vi "Comparison and boolean.VI"() -> ()   [LabVIEW 2019]
panel:
  out "result":bool
  in  "num 3":dbl=20.0
  out "result":bool
  in  "num2":dbl
  out "result":bool
  in  "num 1":dbl=20.0
  out "result":bool
  in  "boolean a":bool
  in  "boolean b":bool
  out "result":bool
  in  "num":dbl=30.0
  # "Comparison"
  # "# For equal to 0 & not equal to 0 comparator"
  # "# For greater than 0 and less than 0 compareator"
  # "# For greater than or equal to 0 and less \nthan or equal to 0"
  # "Boolean"
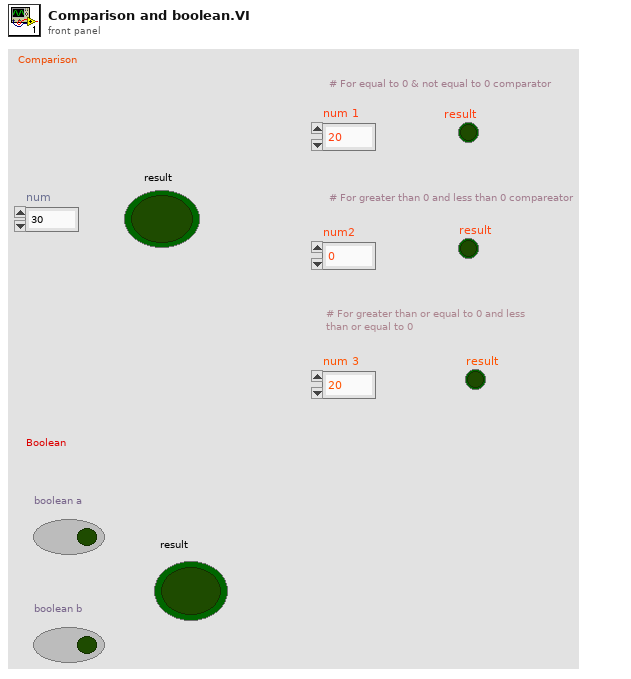
[diagram p1: front panel]
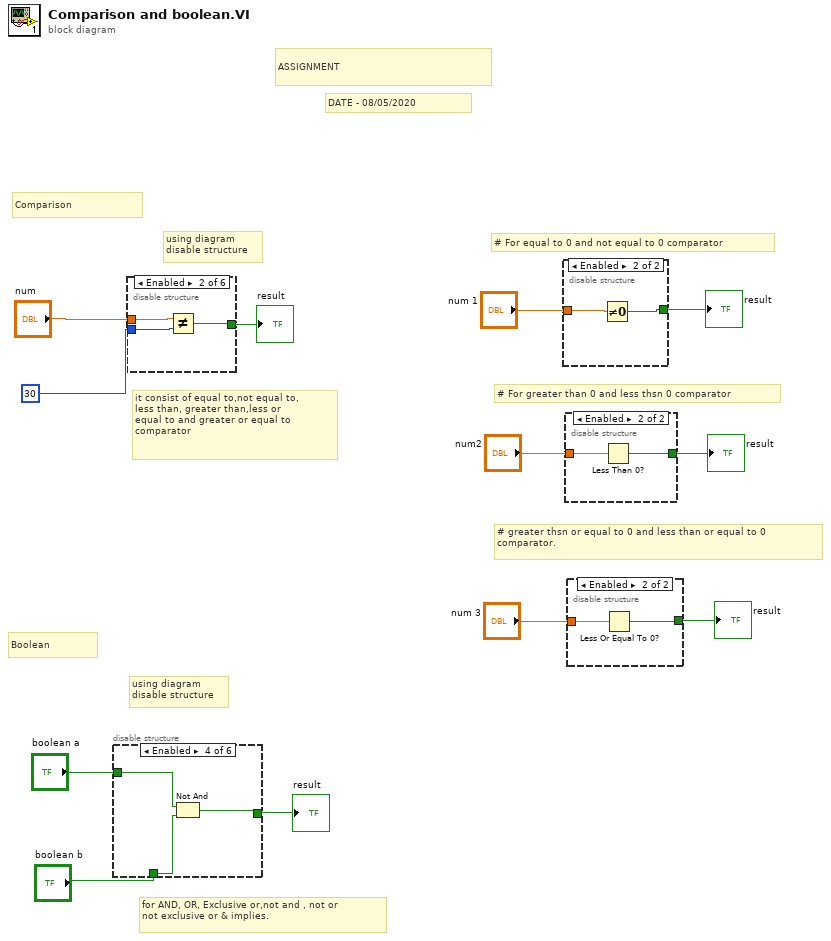
[diagram p0: block diagram]
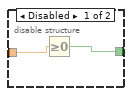
[diagram p2: hidden frame]
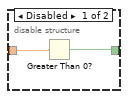
[diagram p3: hidden frame]
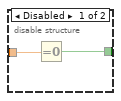
[diagram p4: hidden frame]
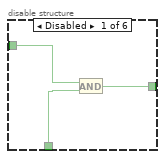
[diagram p5: hidden frame]
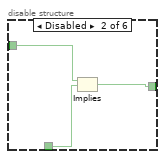
[diagram p6: hidden frame]
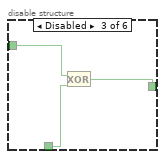
[diagram p7: hidden frame]
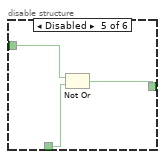
[diagram p8: hidden frame]
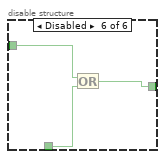
[diagram p9: hidden frame]
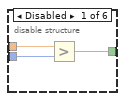
[diagram p10: hidden frame]
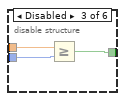
[diagram p11: hidden frame]
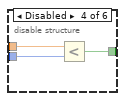
[diagram p12: hidden frame]
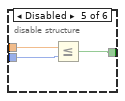
[diagram p13: hidden frame]
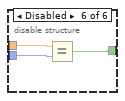
[diagram p14: hidden frame]
diagram:
  # "for AND, OR, Exclusive or,not and , not or\nnot exclusive or & implies."
  # "# greater thsn or equal to 0 and less than or equal to 0\ncomparator."
  # "# For greater than 0 and less thsn 0 comparator"
  # "# For equal to 0 and not equal to 0 comparator"
  # "it consist of equal to,not equal to,\nless than, greater than,less or \nequal to and greater or equal to\ncomparator"
  # "using diagram \ndisable structure"
  # "using diagram \ndisable structure"
  # "DATE - 08/05/2020"
  # "ASSIGNMENT"
  # "Boolean"
  # "Comparison"
  n1 = disable-structure shown="Enabled" {
    disable-tunnel: "boolean a" -> [w15 w18 w21 w24 w27 w30]
    disable-tunnel: "boolean b" -> [w14 w17 w20 w23 w26 w29]
    disable-tunnel: [w13 w16 w19 w22 w25 w28] -> w8
    frame Disabled {
      n2 = And(x=w15, y=w14) -> (x .and. y?=w13:bool)
    }
    frame Disabled {
      n3 = Implies(1:w17, 2:w18) -> (0:w16:bool)
    }
    frame Disabled {
      n4 = Exclusive Or(1:w20, 2:w21) -> (0:w19:bool)
    }
    frame Enabled {
      n5 = Not And(1:w23, 2:w24) -> (0:w22:bool)
    }
    frame Disabled {
      n6 = Not Or(1:w26, 2:w27) -> (0:w25:bool)
    }
    frame Disabled {
      n7 = Or(x=w30, y=w29) -> (x .or. y?=w28:bool)
    }
  }
  "result" <- w8
  n8 = disable-structure shown="Enabled" {
    disable-tunnel: "num" -> [w33 w36 w39 w42 w45 w48]
    disable-tunnel: 30 -> [w32 w35 w38 w41 w44 w47]
    disable-tunnel: [w31 w34 w37 w40 w43 w46] -> w10
    frame Disabled {
      n9 = Greater?(x=w33, y=w32) -> (0:w31:bool)
    }
    frame Enabled {
      n10 = Not Equal?(x=w36, y=w35) -> (x != y?=w34:bool)
    }
    frame Disabled {
      n11 = Greater Or Equal?(x=w39, y=w38) -> (x >= y?=w37:bool)
    }
    frame Disabled {
      n12 = Less?(x=w42, y=w41) -> (x < y?=w40:bool)
    }
    frame Disabled {
      n13 = Less Or Equal?(x=w45, y=w44) -> (x <= y?=w43:bool)
    }
    frame Disabled {
      n14 = Equal?(x=w48, y=w47) -> (x = y?=w46:bool)
    }
  }
  "result" <- w10
  n15 = disable-structure shown="Enabled" {
    disable-tunnel: "num 1" -> [w50 w52]
    disable-tunnel: [w49 w51] -> w5
    frame Disabled {
      n16 = Equal To 0?(x=w50) -> (x = 0?=w49:bool)
    }
    frame Enabled {
      n17 = Not Equal To 0?(x=w52) -> (x != 0?=w51:bool)
    }
  }
  "result" <- w5
  n18 = disable-structure shown="Enabled" {
    disable-tunnel: "num2" -> [w54 w56]
    disable-tunnel: [w53 w55] -> w3
    frame Disabled {
      n19 = Greater Than 0?(x=w54) -> (x > 0?=w53:bool)
    }
    frame Enabled {
      n20 = Less Than 0?(x=w56) -> (x < 0?=w55:bool)
    }
  }
  "result" <- w3
  n21 = disable-structure shown="Enabled" {
    disable-tunnel: "num 3" -> [w58 w60]
    disable-tunnel: [w57 w59] -> w1
    frame Disabled {
      n22 = Greater Or Equal To 0?(x=w58) -> (x >= 0?=w57:bool)
    }
    frame Enabled {
      n23 = Less Or Equal To 0?(x=w60) -> (x <= 0?=w59:bool)
    }
  }
  "result" <- w1
